vi "Prepare Panel GObject for Move.vi"(6 "Reference Text to Append (\" Ref\")":string=" Ref", 8 "error in (no error)":errorcluster, 9 "Add as Reference?":bool, 11 "GObject in":refnum<vi>) -> (0 "error out":errorcluster, 1 "Updated Add as Reference?":bool, 2 "Label.Text":string, 3 "GObject out":refnum<vi>)   [LabVIEW 2020, in "Add to Private Data.lvlib"]
uses:
  Add to Private Data.lvlib
  <vilib>/ErrorRing/Error Ring.xnode
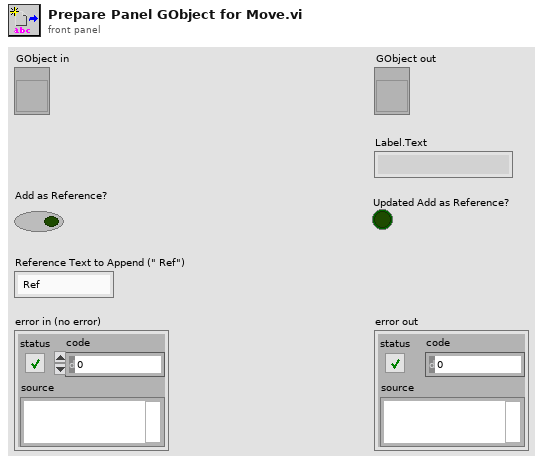
[diagram p1: front panel]
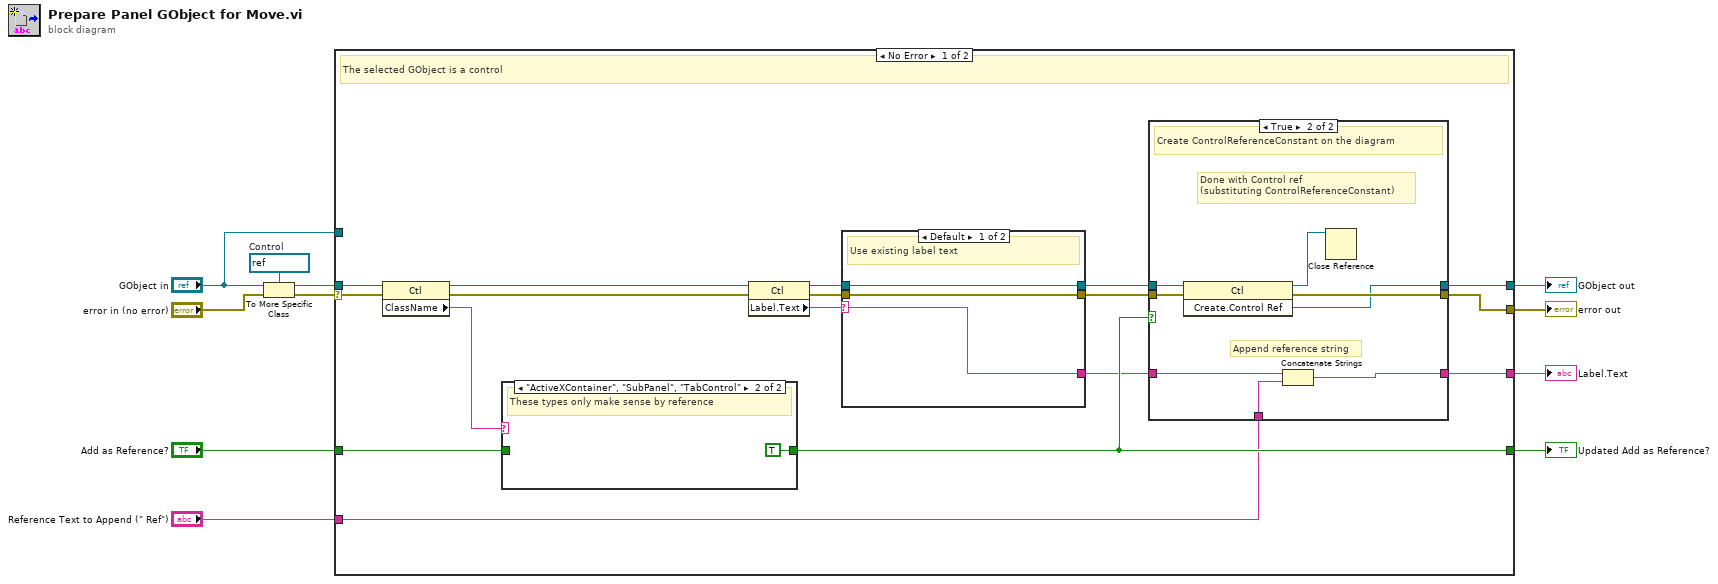
[diagram p0: block diagram]
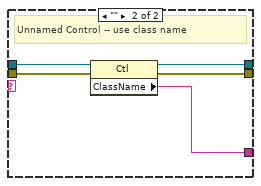
[diagram p3: hidden frame]
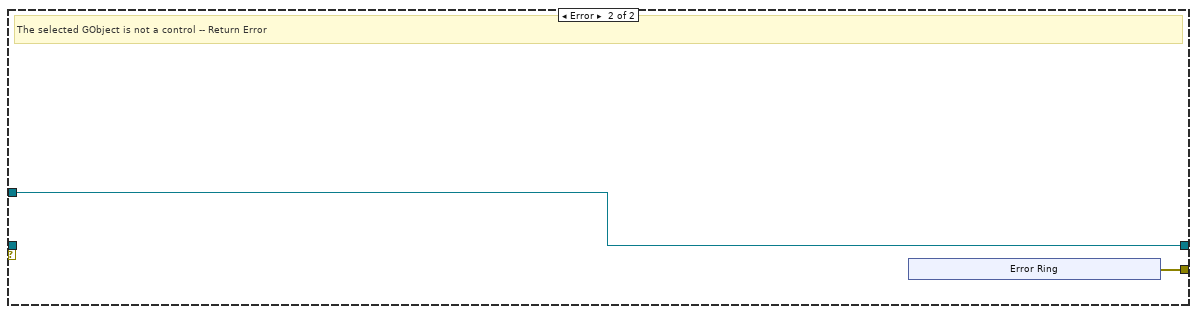
[diagram p5: hidden frame]
diagram:
  w5 = refnum<vi> refnum  # Control
  n1 = To More Specific Class(target class=w5, reference="GObject in", error in="error in (no error)") -> (specific class reference=w6:refnum<vi>, error out=w3:errorcluster)
  n2 = case shown="No Error" w3 {
    selector: w3 -> [w23 _]
    tunnel: [w28 w50] -> w11
    tunnel: [w27 w51] -> w10
    tunnel: "Add as Reference?" -> [w16 _]
    tunnel: "Reference Text to Append (\" Ref\")" -> [w12 _]
    tunnel: [w15 _] -> w7
    tunnel: w6 -> [w24 _]
    tunnel: "GObject in" -> [_ w51]
    tunnel: [w13 _] -> w1
    frame No Error {
      # "The selected GObject is a control"
      n3 = property class="Ctl"(reference=w24, error in=w23) -> (reference out=w26:refnum<vi>, error out=w25:errorcluster, "ClassName"=w17:string)
      n4 = case shown="\"ActiveXContainer\", \"SubPanel\", \"TabControl\"" w17 {
        tunnel: w16 -> [w29 _]
        tunnel: [w29 TRUE ("Add as Reference?")] -> w15
        frame Default {
          # "Do not modify user's by-ref/by-value choice"
        }
        frame "ActiveXContainer", "SubPanel", "TabControl" {
          # "These types only make sense by reference"
        }
      }
      n5 = property class="Ctl"(reference=w26, error in=w25) -> (reference out=w20:refnum<vi>, error out=w21:errorcluster, "Label.Text"=w22:string)
      n6 = case shown="Default" w22 {
        selector: w22 -> [w32 _]
        tunnel: w20 -> [w31 w38]
        tunnel: [w31 w37] -> w19
        tunnel: w21 -> [w33 w36]
        tunnel: [w33 w35] -> w18
        tunnel: [w32 w34] -> w14
        frame Default {
          # "Use existing label text"
        }
        frame "" {
          # "Unnamed Control -- use class name"
          n7 = property class="Ctl"(reference=w38, error in=w36) -> (reference out=w37:refnum<vi>, error out=w35:errorcluster, "ClassName"=w34:string)
        }
      }
      n8 = case shown="True" w15 {
        tunnel: [w41 w49] -> w28
        tunnel: [w40 w48] -> w27
        tunnel: w19 -> [w40 w47]
        tunnel: w18 -> [w41 w46]
        tunnel: w14 -> [w39 w44]
        tunnel: [w39 w43] -> w13
        tunnel: w12 -> [_ w42]
        frame False {
          # "Adding as value control -- do nothing"
        }
        frame True {
          # "Append reference string"
          # "Done with Control ref\n(substituting ControlReferenceConstant)"
          # "Create ControlReferenceConstant on the diagram"
          n9 = invoke class="Ctl" method="Create.Control Ref"(reference=w47, error in=w46) -> (reference out=w45:refnum<vi>, error out=w49:errorcluster, "Create Control Ref"=w48:refnum<vi>)  [unwired: 1 in]
          n10 = Concatenate Strings(w44, w42) -> (w43:string)
          n11 = Close Reference(reference=w45) -> ()  [unwired: 1 in, 1 out]
        }
      }
    }
    frame Error {
      # "The selected GObject is not a control -- Return Error"
      n12 = xnode "Error Ring"() -> ("error out"=w50:errorcluster)
    }
  }
  "error out" <- w11
  "GObject out" <- w10
  "Label.Text" <- w1
  "Updated Add as Reference?" <- w7
